vi "Read Buffer.vi"(11 "Buffer Download Controller in":refnum<class "Buffer Download Controller.lvclass">) -> (2 "buffer":u8[](array[numeric]), 3 "Buffer Download Controller out":refnum<class "Buffer Download Controller.lvclass">)   [LabVIEW 2020, in "NI_SFTP.lvlib" / "Buffer Download Controller.lvclass"]
uses:
  <vilib>/net/SFTP/API/Support/Download/Buffer/Buffer Download Controller.lvclass
  <vilib>/net/SFTP/API/Support/Download/Buffer/Buffer Download Controller.lvclass/Buffer Download Controller.ctl
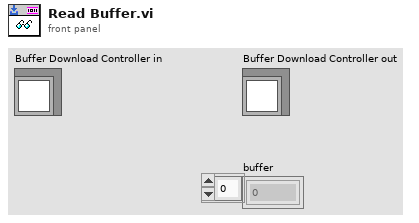
[diagram p1: front panel]
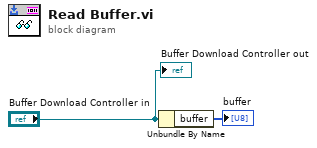
[diagram p0: block diagram]
diagram:
  n1 = Unbundle By Name("Buffer Download Controller in") -> ("buffer"=→"buffer":u8[])
  "Buffer Download Controller out" <- "Buffer Download Controller in"
